vi "Bus Interface.vi"(0 "niInstr AXI4-Lite - FXP32 address - fxp32 data v1 FPGA in":refnum<class "niInstr AXI4-Lite - FXP32 Address - FXP32 Data v1 FPGA.lvclass">, 1 "abort":bool, 5 "address space.lvclass:address space instruction in":T2, 9 "input valid (instruction)":bool) -> (6 "response out":T1, 10 "done":bool, 14 "ready for input":bool)   [LabVIEW 2015, in "niInstr AXI4-Lite - FXP32 Address - FXP32 Data v1 FPGA.lvclass"]
doc: "Manages the mapping between AXI4-Lite and the Instruction Framework and performs the bus transactions.\n\n<B>Input Parameters</B>\n\n<B>niInstr AXI4-Lite - FXP32 address - fxp32 data v1 FPGA in</B> is a reference to the class used to communicate.\n\n<B>abort</B> aborts the current data transaction. Currently unsupported.\n\n<B>address space.lvclass:address space instruction in</B> specifies the instruction to be written.\n\n<B>address space.lvclass:address space instruction in.address</B> specifies the address of the instruction to be written.\n\n<B>address space.lvclass:address space instruction in.data</B> specifies the instruction data to be written.\n\n<B>address space.lvclass:address space instruction in.read</B> is true for Read instructions and false for Write instructions.\n\n<B>input valid (instruction)</B> is true if the instruction on the current clock cycle is valid.\n\n<B>Output Parameters</B>\n\n<B>response out</B> is the response from the bus. This parameter is valid only if 'done' returns true.\n\n<B>response out.data</B> is the data of the response.\n\n<B>response out.error</B> is true if there was an error as part of the response.\n\n<B>done</B> indicates whether the received 'response out' is valid.\n\n<B>ready for input</B> indicates whether the bus is ready to accept more data."
uses:
  <instrlib>/_niInstr/CLIP Adapters/v1/FPGA/AXI4-Lite/FXP32 Address - FXP32 Data/niInstr AXI4-Lite - FXP32 Address - FXP32 Data v1 FPGA.lvclass
  <instrlib>/_niInstr/Instruction Framework/v1/FPGA/Interfaces/Address Space/Address Space Instruction.ctl
  <instrlib>/_niInstr/Instruction Framework/v1/FPGA/Typedefs/Response.ctl
  <instrlib>/_niInstr/CLIP Adapters/v1/FPGA/AXI4-Lite/FXP32 Address - FXP32 Data/niInstr AXI4-Lite - FXP32 Address - FXP32 Data v1 FPGA.lvclass/niInstr AXI4-Lite - FXP32 Address - FXP32 Data v1 FPGA.ctl
  <instrlib>/_niInstr/CLIP Adapters/v1/FPGA/AXI4-Lite/Address Space/Protected/AXI4-Lite State Machine State.ctl
  <instrlib>/_niInstr/CLIP Adapters/v1/FPGA/AXI4-Lite/Address Space/Protected/AXI4-Lite Read State.ctl
  <instrlib>/_niInstr/CLIP Adapters/v1/FPGA/AXI4-Lite/Address Space/Protected/AXI4-Lite Write State.ctl
  <vilib>/rvi/eio/common/nirviEmuTemplateMethod_errors.vi
  <vilib>/eio/EIONode/EIONode.xnode
  <instrlib>/_niInstr/CLIP Adapters/v1/FPGA/AXI4-Lite/Address Space/niInstr AXI4-Lite Address Space v1 FPGA.lvclass
  <instrlib>/_niInstr/Instruction Framework/v1/FPGA/Typedefs/niInstr Instruction Framework v1 FPGA.lvlib
  <instrlib>/_niInstr/Instruction Framework/v1/FPGA/Interfaces/Address Space/Address Space.lvclass
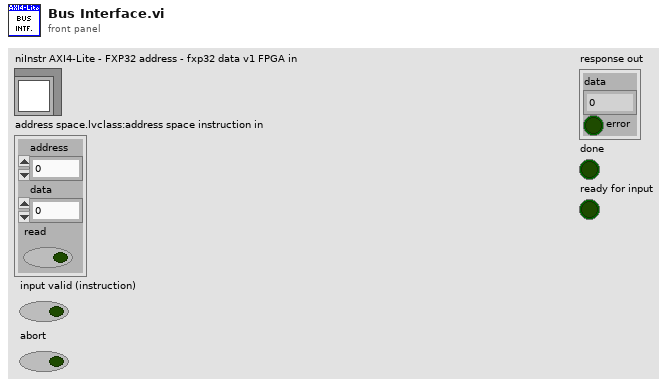
[diagram p1: front panel]
types:
  T1 = typedef "niInstr Instruction Framework v1 FPGA.lvlib/Response.ctl" = cluster{"data":u64, "error":bool}
  T2 = typedef "niInstr Instruction Framework Interfaces v1 FPGA.lvlib/Address Space.lvclass/Address Space Instruction.ctl" = cluster{"address":u32, "data":u64, "read":bool}
  T3 = typedef "niInstr AXI4-Lite Address Space v1 FPGA.lvclass/AXI4-Lite Write State.ctl" = enum16{"Send Write Address and Write Data", "Receive Write Response"}
  T4 = typedef "niInstr AXI4-Lite Address Space v1 FPGA.lvclass/AXI4-Lite Read State.ctl" = enum16{"Send Read Address", "Receive Read Data"}
  T5 = typedef "niInstr AXI4-Lite Address Space v1 FPGA.lvclass/AXI4-Lite State Machine State.ctl" = enum16{"Initialize", "Wait for Instruction", "Read", "Write"}
  T6 = typedef "AXI4-Lite Address Space.lvclass/AXI4-Lite State Machine State.ctl" = enum16{"Initialize", "Wait for Instruction", "Read", "Write"}
  T7 = typedef "AXI4-Lite Address Space.lvclass/AXI4-Lite Read State.ctl" = enum16{"Send Read Address", "Receive Read Data"}
  T8 = typedef "AXI4-Lite Address Space.lvclass/AXI4-Lite Write State.ctl" = enum16{"Send Write Address and Write Data", "Receive Write Response"}
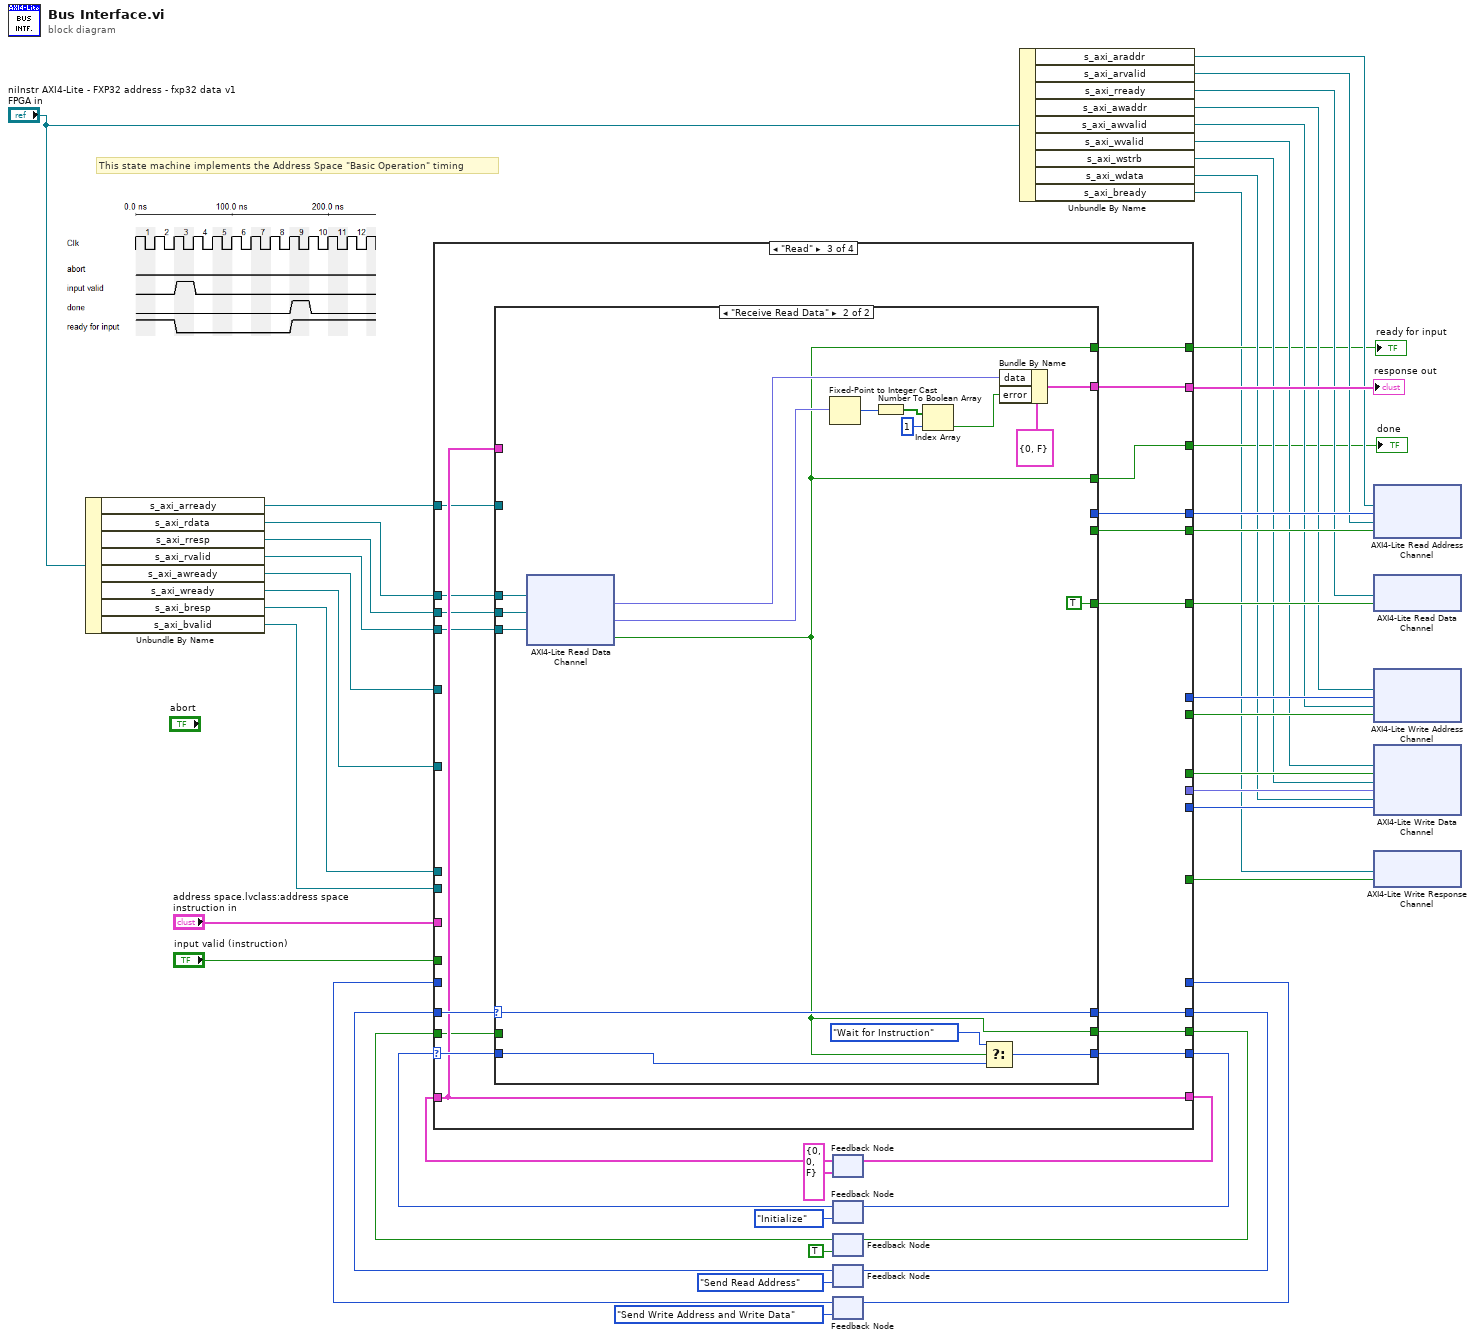
[diagram p0: block diagram]
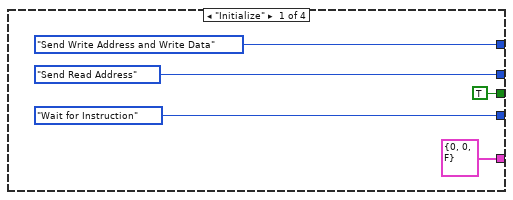
[diagram p2: hidden frame]
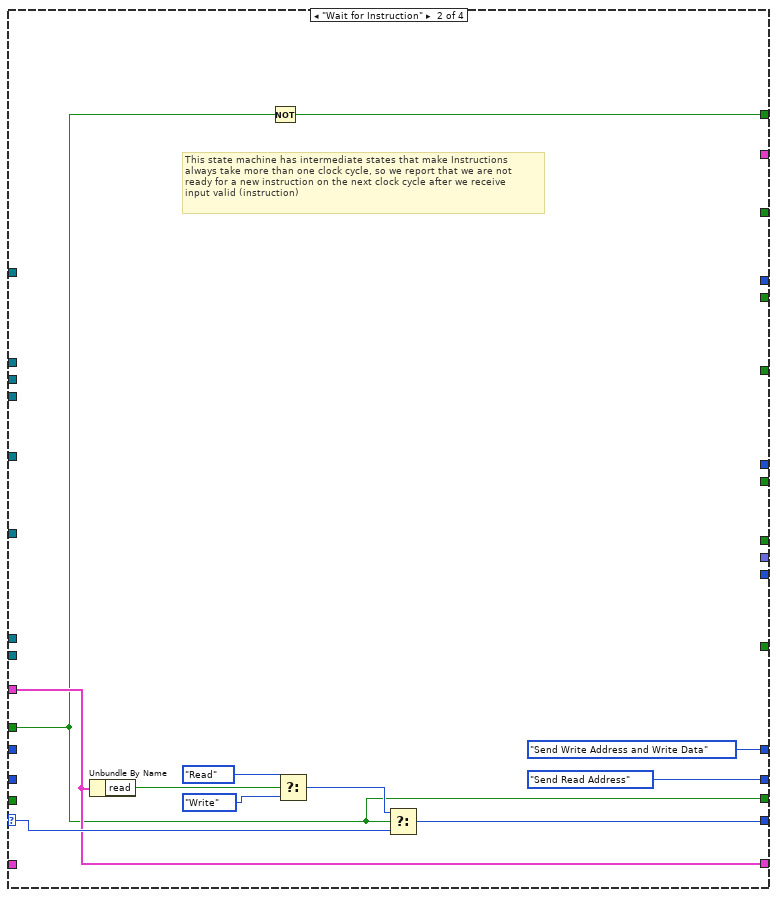
[diagram p3: hidden frame]
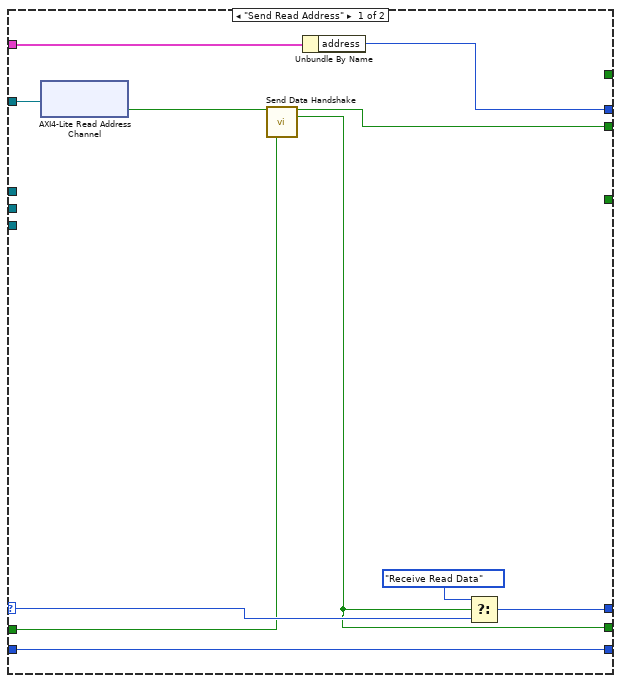
[diagram p4: hidden frame]
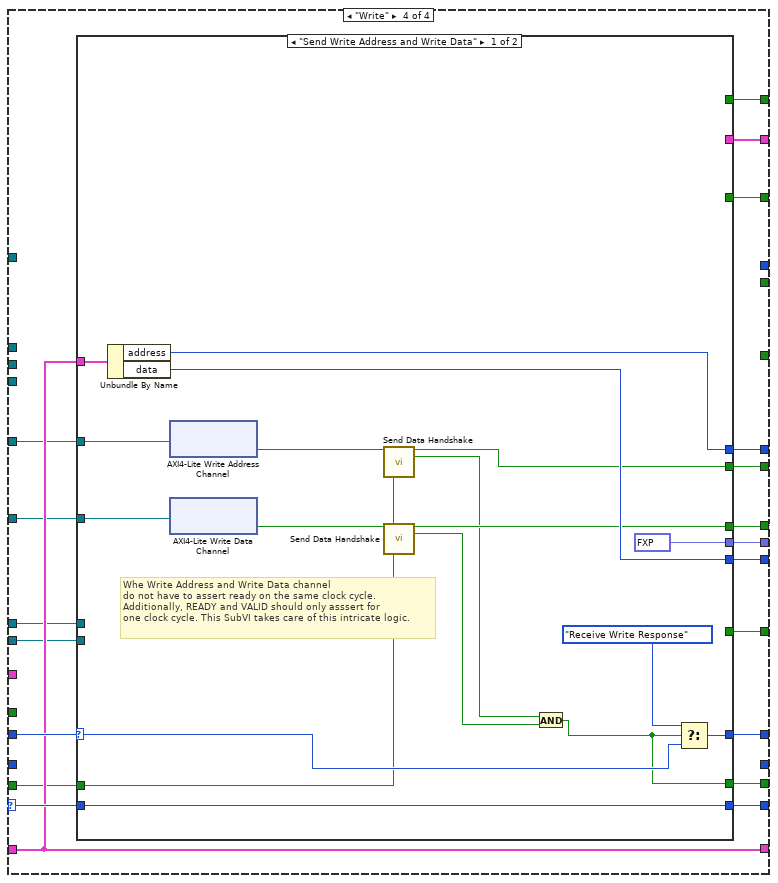
[diagram p5: hidden frame]
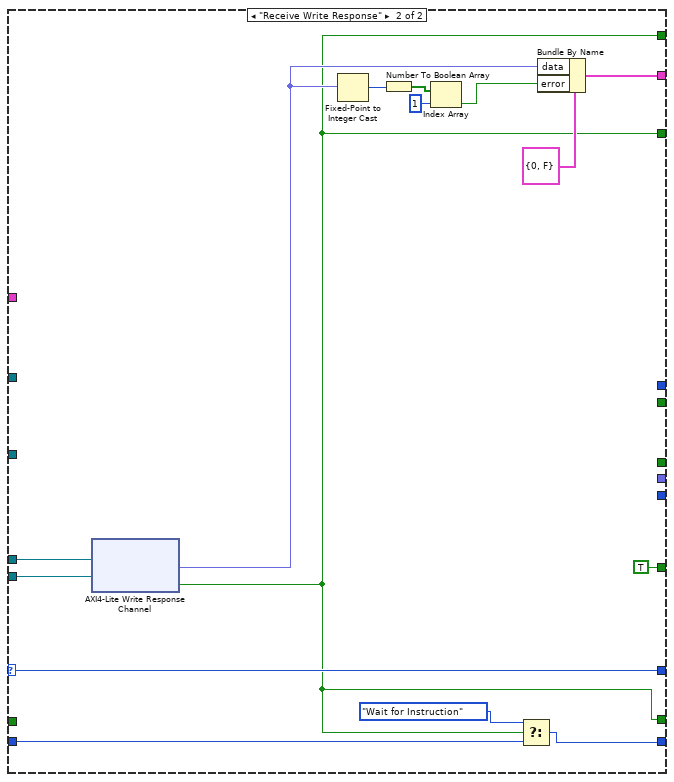
[diagram p6: hidden frame]
diagram:
  # "This state machine implements the Address Space \"Basic Operation\" timing"
  n1 = Unbundle By Name("niInstr AXI4-Lite - FXP32 address - fxp32 data v1 FPGA in") -> ("s_axi_arready"=w16:refnum<k21>, "s_axi_rdata"=w17:refnum<k21>, "s_axi_rresp"=w18:refnum<k21>, "s_axi_rvalid"=w19:refnum<k21>, "s_axi_awready"=w7:refnum<k21>, "s_axi_wready"=w15:refnum<k21>, "s_axi_bresp"=w14:refnum<k21>, "s_axi_bvalid"=w13:refnum<k21>)
  n2 = feedback #1(T2 {"address"=0, "data"=0, "read"=FALSE} ("instruction")) -> (w42:T2)
  n3 = feedback #2(AXI4-Lite_State_Machine_State."Initialize") -> (w5:T6)
  n4 = feedback #3(TRUE) -> (w3:bool)
  n5 = feedback #4(AXI4-Lite_Read_State."Send Read Address") -> (w44:T7)
  n6 = feedback #5(AXI4-Lite_Write_State."Send Write Address and Write Data" ("Enum")) -> (w43:T8)
  n7 = case shown="\"Read\"" w5 {
    selector: w5 -> [_ w60 w77 w124]
    tunnel: "address space.lvclass:address space instruction in" -> [_ w56 _ _]
    tunnel: "input valid (instruction)" -> [_ w53 _ _]
    tunnel: [T2 {"address"=0, "data"=0, "read"=FALSE} ("instruction") w56 w72 w116] -> w45
    tunnel: w42 -> [_ _ w72 w116]
    tunnel: [AXI4-Lite_State_Machine_State."Wait for Instruction" w59 w78 w123] -> w6
    tunnel: [AXI4-Lite_Read_State."Send Read Address" AXI4-Lite_Read_State."Send Read Address" w79 _] -> w9
    tunnel: w44 -> [_ _ w80 _]
    tunnel: [_ _ w76 w125] -> w12
    tunnel: [_ _ w75 w126] -> w46
    tunnel: [AXI4-Lite_Write_State."Send Write Address and Write Data" ("Enum") AXI4-Lite_Write_State."Send Write Address and Write Data" ("Enum") _ w127] -> w8
    tunnel: w43 -> [_ _ _ w128]
    tunnel: [_ _ _ w122] -> w37
    tunnel: [_ _ _ w121] -> w32
    tunnel: [_ _ w74 _] -> w36
    tunnel: [_ _ w73 _] -> w35
    tunnel: [_ _ _ w120] -> w34
    tunnel: [_ _ w71 _] -> w33
    tunnel: [_ _ _ w119] -> w31
    tunnel: [_ _ _ w118] -> w30
    tunnel: [_ _ _ w117] -> w29
    tunnel: w19 -> [_ _ w70 _]
    tunnel: w18 -> [_ _ w69 _]
    tunnel: w17 -> [_ _ w68 _]
    tunnel: w16 -> [_ _ w67 _]
    tunnel: w7 -> [_ _ _ w115]
    tunnel: w15 -> [_ _ _ w114]
    tunnel: w14 -> [_ _ _ w113]
    tunnel: w13 -> [_ _ _ w112]
    tunnel: [_ w54 w66 w111] -> w11
    tunnel: w3 -> [_ _ w64 w110]
    tunnel: [TRUE ("I/O Item") w53 w65 w109] -> w4
    frame "Initialize" {
    }
    frame "Wait for Instruction" {
      # "This state machine has intermediate states that make Instructions \nalways take more than one clock cycle, so we report that we are not \nready for a new instruction on the next clock cycle after we receive\ninput valid (instruction)"
      n8 = Unbundle By Name(w56) -> ("read"=w63:bool)
      n9 = Not(x=w53) -> (.not. x?=w54:bool)
      n10 = Select(t=AXI4-Lite_State_Machine_State."Read", s=w63, f=AXI4-Lite_State_Machine_State."Write") -> (s? t:f=w62:T5)
      n11 = Select(t=w62, s=w53, f=w60) -> (s? t:f=w59:T6)
    }
    frame "Read" {
      n12 = case shown="\"Receive Read Data\"" w80 {
        selector: w80 -> [w91 w108]
        tunnel: w72 -> [w86 _]
        tunnel: [w88 w108] -> w79
        tunnel: [w83 _] -> w74
        tunnel: [w89 w107] -> w78
        tunnel: w77 -> [w89 w106]
        tunnel: [_ w93] -> w76
        tunnel: [_ w104] -> w75
        tunnel: [_ TRUE ("I/O Item")] -> w73
        tunnel: [w87 _] -> w71
        tunnel: w70 -> [_ w96]
        tunnel: w69 -> [_ w95]
        tunnel: w68 -> [_ w94]
        tunnel: w67 -> [w85 _]
        tunnel: [_ w93] -> w66
        tunnel: [w81 w93] -> w65
        tunnel: w64 -> [w82 _]
        frame "Send Read Address" {
          n13 = xnode "AXI4-Lite Read Address Channel"("FPGA I/O In"=w85) -> ("I/O Item"=w84:bool)  [unwired: 1 out]
          n14 = call <instrlib>:"Send Data Handshake.vi"("READY"=w84, "first iteration in this state?"=w82) -> ("VALID"=w83:bool, "done?"=w81:bool)  [unwired: 12 in]
          n15 = Unbundle By Name(w86) -> ("address"=w87:u32)
          n16 = Select(t=AXI4-Lite_Read_State."Receive Read Data", s=w81, f=w91) -> (s? t:f=w88:T7)
        }
        frame "Receive Read Data" {
          n17 = xnode "AXI4-Lite Read Data Channel"("FPGA I/O In"=w94, "FPGA I/O In"=w95, "FPGA I/O In"=w96) -> ("I/O Item"=w103:fxp<+,32,32>, "I/O Item"=w99:fxp<+,2,2>, "I/O Item"=w93:bool)  [unwired: 3 out]
          n18 = Fixed-Point to Integer Cast(1:w99) -> (0:w101:u8)
          n19 = Number To Boolean Array(number=w101) -> (Boolean array=w100:bool[])
          n20 = Index Array(array=w100, index=1) -> (element=w98:bool)
          n21 = Select(t=AXI4-Lite_State_Machine_State."Wait for Instruction", s=w93, f=w106) -> (s? t:f=w107:T6)
          n22 = Bundle By Name(cluster=T1 {"data"=0, "error"=FALSE} ("response"), "data"=w103, "error"=w98) -> (w104:T1)
        }
      }
    }
    frame "Write" {
      n23 = case shown="\"Send Write Address and Write Data\"" w128 {
        selector: w128 -> [w146 w156]
        tunnel: [w133 _] -> w122
        tunnel: [w132 _] -> w121
        tunnel: [w145 w156] -> w127
        tunnel: w116 -> [w143 _]
        tunnel: [_ w160] -> w126
        tunnel: [_ w148] -> w125
        tunnel: w124 -> [w142 w159]
        tunnel: [w142 w158] -> w123
        tunnel: [_ TRUE ("I/O Item")] -> w120
        tunnel: [fxp<+,4,4> 15.0 ("blk_mem_gen_v7_3 1\\s_axi_wstrb") _] -> w119
        tunnel: [w140 _] -> w118
        tunnel: [w139 _] -> w117
        tunnel: w115 -> [w138 _]
        tunnel: w114 -> [w137 _]
        tunnel: w113 -> [_ w150]
        tunnel: w112 -> [_ w149]
        tunnel: [_ w148] -> w111
        tunnel: w110 -> [w136 _]
        tunnel: [w129 w148] -> w109
        frame "Send Write Address and Write Data" {
          # "Whe Write Address and Write Data channel\ndo not have to assert ready on the same clock cycle.\nAdditionally, READY and VALID should only asssert for \none clock cycle. This SubVI takes care of this intricate logic."
          n24 = Unbundle By Name(w143) -> ("address"=w140:u32, "data"=w139:u64)
          n25 = xnode "AXI4-Lite Write Address Channel"("FPGA I/O In"=w138) -> ("I/O Item"=w135:bool)  [unwired: 1 out]
          n26 = xnode "AXI4-Lite Write Data Channel"("FPGA I/O In"=w137) -> ("I/O Item"=w134:bool)  [unwired: 1 out]
          n27 = call <instrlib>:"Send Data Handshake.vi"("READY"=w135, "first iteration in this state?"=w136) -> ("VALID"=w133:bool, "done?"=w131:bool)  [unwired: 12 in]
          n28 = call <instrlib>:"Send Data Handshake.vi"("READY"=w134, "first iteration in this state?"=w136) -> ("VALID"=w132:bool, "done?"=w130:bool)  [unwired: 12 in]
          n29 = And(x=w131, y=w130) -> (x .and. y?=w129:bool)
          n30 = Select(t=AXI4-Lite_Write_State."Receive Write Response", s=w129, f=w146) -> (s? t:f=w145:T8)
        }
        frame "Receive Write Response" {
          n31 = xnode "AXI4-Lite Write Response Channel"("FPGA I/O In"=w150, "FPGA I/O In"=w149) -> ("I/O Item"=w152:fxp<+,2,2>, "I/O Item"=w148:bool)  [unwired: 2 out]
          n32 = Fixed-Point to Integer Cast(1:w152) -> (0:w155:u8)
          n33 = Number To Boolean Array(number=w155) -> (Boolean array=w154:bool[])
          n34 = Index Array(array=w154, index=1) -> (element=w151:bool)
          n35 = Select(t=AXI4-Lite_State_Machine_State."Wait for Instruction", s=w148, f=w159) -> (s? t:f=w158:T6)
          n36 = Bundle By Name(cluster=T1 {"data"=0, "error"=FALSE} ("response"), "data"=w152, "error"=w151) -> (w160:T1)
        }
      }
    }
  }
  "response out" <- w46
  "done" <- w12
  "ready for input" <- w11
  n37 = feedback-in #1(w45) -> ()
  n38 = feedback-in #2(w6) -> ()
  n39 = feedback-in #3(w4) -> ()
  n40 = feedback-in #4(w9) -> ()
  n41 = feedback-in #5(w8) -> ()
  n42 = Unbundle By Name("niInstr AXI4-Lite - FXP32 address - fxp32 data v1 FPGA in") -> ("s_axi_araddr"=w28:refnum<k21>, "s_axi_arvalid"=w27:refnum<k21>, "s_axi_rready"=w26:refnum<k21>, "s_axi_awaddr"=w25:refnum<k21>, "s_axi_awvalid"=w24:refnum<k21>, "s_axi_wvalid"=w23:refnum<k21>, "s_axi_wstrb"=w22:refnum<k21>, "s_axi_wdata"=w21:refnum<k21>, "s_axi_bready"=w1:refnum<k21>)
  n43 = xnode "AXI4-Lite Read Address Channel"("I/O Item"=w33, "FPGA I/O In"=w28, "I/O Item"=w36, "FPGA I/O In"=w27) -> ()  [unwired: 2 out]
  n44 = xnode "AXI4-Lite Read Data Channel"("I/O Item"=w35, "FPGA I/O In"=w26) -> ()  [unwired: 1 out]
  n45 = xnode "AXI4-Lite Write Address Channel"("I/O Item"=w30, "FPGA I/O In"=w25, "I/O Item"=w37, "FPGA I/O In"=w24) -> ()  [unwired: 2 out]
  n46 = xnode "AXI4-Lite Write Data Channel"("I/O Item"=w32, "FPGA I/O In"=w23, "I/O Item"=w31, "FPGA I/O In"=w22, "I/O Item"=w29, "FPGA I/O In"=w21) -> ()  [unwired: 3 out]
  n47 = xnode "AXI4-Lite Write Response Channel"("I/O Item"=w34, "FPGA I/O In"=w1) -> ()  [unwired: 1 out]
